vi "Event Notification.Status Message with Error In.vi"(4 "Display":bool=TRUE, 5 "FWD":bool, 6 "Log":bool=TRUE, 7 "Level":T2 caption="Level(Normal)", 8 "Error":errorcluster, 9 "Type":T1, 10 "Message":string, 11 "Event Notification in":refnum<class "Event Notification.lvclass">) -> ()   [LabVIEW 2024, in "EQMF.lvlib" / "Event Log.lvlib" / "Event Notification.lvclass"]
uses:
  Event Notification.lvclass
  Event Log.Log Level.ctl
  Event Log.Notification Type.ctl
  Event Notification.lvclass/Event Notification.ctl
  Event Log.lvlib
  Queues/Queue Utils.lvlib
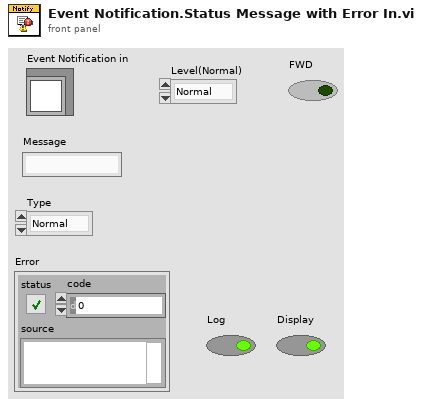
[diagram p1: front panel]
types:
  T1 = typedef "EQMF.lvlib/Event Log.lvlib/Event Log.Notification Type.ctl" = enum16{"Normal", "Warning", "Error", "Success"}
  T2 = typedef "EQMF.lvlib/Event Log.lvlib/Event Log.Log Level.ctl" = enum16{"Normal", "Verbose", "Debug0", "Debug1", "Debug2"}
  T3 = cluster{"Normal":u32, "Warning":u32, "Error":u32, "Success":u32}
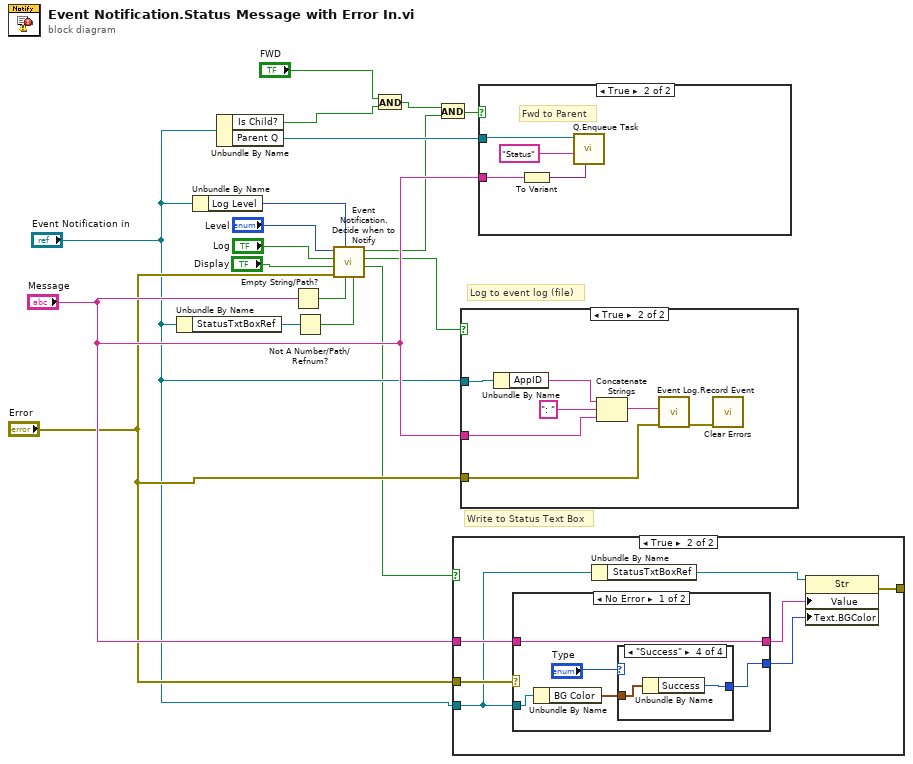
[diagram p0: block diagram]
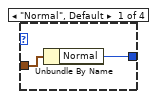
[diagram p4: hidden frame]
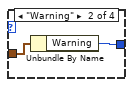
[diagram p5: hidden frame]
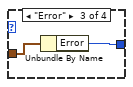
[diagram p6: hidden frame]
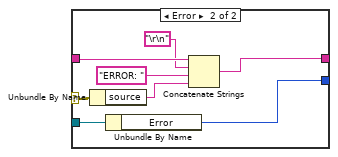
[diagram p7: hidden frame]
diagram:
  # "Write to Status Text Box"
  # "Log to event log (file)"
  n1 = Unbundle By Name("Event Notification in") -> ("StatusTxtBoxRef"=w16:refnum<vi>)
  n2 = Unbundle By Name("Event Notification in") -> ("Log Level"=w11:T2)
  n3 = Unbundle By Name("Event Notification in") -> ("Is Child?"=w2:bool, "Parent Q"=w17:refnum<queue>)
  n4 = Empty String/Path?(string/path="Message") -> (empty?=w18:bool)
  n5 = Not A Number/Path/Refnum?(number/path/refnum=w16) -> (NaN/Path/Refnum?=w10:bool)
  n6 = call "Event Notification.Decide when to Notify.vi"("IsNotControlRef"=w10, "IsEmptyStr"=w18, "Sys Level"=w11, "error in"="Error", "Display"="Display", "Log"="Log", "Level"="Level") -> ("Display"=w4:bool, "Log"=w8:bool, "Fwd to Parent"=w9:bool)  [unwired: 2 in]
  n7 = And(x="FWD", y=w2) -> (x .and. y?=w1:bool)
  n8 = And(x=w1, y=w9) -> (x .and. y?=w15:bool)
  n9 = case shown="True" w4 {
    tunnel: "Message" -> [_ w22]
    tunnel: [_ w25] -> _
    tunnel: "Error" -> [_ w24]
    tunnel: "Event Notification in" -> [_ w20]
    frame False {
    }
    frame True {
      n10 = case shown="No Error" w24 {
        selector: w24 -> [_ w41]
        tunnel: [w30 w39] -> w23
        tunnel: w22 -> [w30 w44]
        tunnel: w20 -> [w29 w46]
        tunnel: [w26 w45] -> w21
        frame No Error {
          n11 = Unbundle By Name(w29) -> ("BG Color"=w27:T3)
          n12 = case shown="\"Success\"" "Type" {
            tunnel: w27 -> [w32 w34 w36 w38]
            tunnel: [w31 w33 w35 w37] -> w26
            frame "Normal", Default {
              n13 = Unbundle By Name(w32) -> ("Normal"=w31:u32)
            }
            frame "Warning" {
              n14 = Unbundle By Name(w34) -> ("Warning"=w33:u32)
            }
            frame "Error" {
              n15 = Unbundle By Name(w36) -> ("Error"=w35:u32)
            }
            frame "Success" {
              n16 = Unbundle By Name(w38) -> ("Success"=w37:u32)
            }
          }
        }
        frame Error {
          n17 = Unbundle By Name(w41) -> ("source"=w40:string)
          n18 = Unbundle By Name(w46) -> ("Error"=w45:u32)
          n19 = Concatenate Strings(w44, "\r\n", "ERROR: ", w40) -> (w39:string)
        }
      }
      n20 = Unbundle By Name(w20) -> ("StatusTxtBoxRef"=w19:refnum<vi>)
      n21 = property class="Str"(reference=w19, "Value"=w23, "Text.BGColor"=w21) -> (error out=w25:errorcluster)  [unwired: 1 in, 1 out]
    }
  }
  n22 = case shown="True" w8 {
    tunnel: "Message" -> [_ w50]
    tunnel: "Event Notification in" -> [_ w53]
    tunnel: "Error" -> [_ w48]
    frame False {
    }
    frame True {
      n23 = Unbundle By Name(w53) -> ("AppID"=w52:string)
      n24 = Concatenate Strings(w52, ": ", w50) -> (w49:string)
      n25 = call "Event Log.Record Event.vi"("error in"=w48, "Message"=w49) -> ("error out"=w47:errorcluster)  [unwired: 9 in]
      n26 = call <vilib>:"Clear Errors.vi"("error in (no error)"=w47) -> ()  [unwired: 5 in, 2 out]
    }
  }
  n27 = case shown="True" w15 {
    tunnel: w17 -> [_ w57]
    tunnel: "Message" -> [_ w54]
    frame False {
    }
    frame True {
      # "Fwd to Parent"
      n28 = To Variant(anything=w54) -> (Variant=w55:variant)
      n29 = call "Q.Enqueue Task.vi"("Data1"=w55, "Task Name"="Status", "Q In"=w57) -> ()  [unwired: 7 in, 2 out]
    }
  }
